vi "Write Next Row (First Column).vi"(8 "error in (no error)":errorcluster, 10 "Next Row":i32, 11 "PQ Result  in":refnum<class "PQ Result.lvclass">) -> (0 "error out":errorcluster, 3 "PQ Result  out":refnum<class "PQ Result.lvclass">)   [LabVIEW 2013, in "PQ Result.lvclass"]
uses:
  PQ Result.lvclass
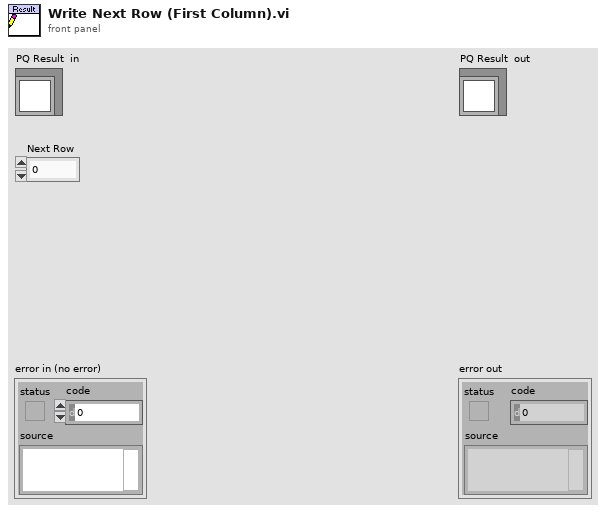
[diagram p1: front panel]
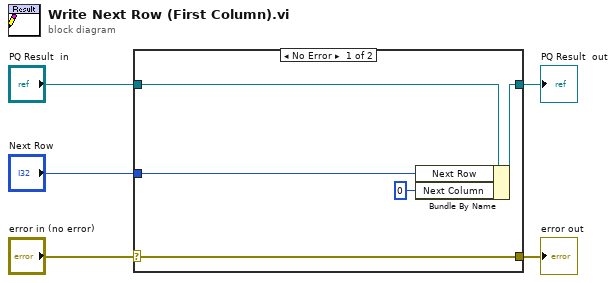
[diagram p0: block diagram]
diagram:
  n1 = case shown="No Error" "error in (no error)" {
    selector: "error in (no error)" -> [w10 w11]
    tunnel: [w10 w11] -> w4
    tunnel: [w8 w12] -> w2
    tunnel: "PQ Result  in" -> [w9 w12]
    tunnel: "Next Row" -> [w7 _]
    frame No Error {
      n2 = Bundle By Name(cluster=w9, "Next Row"=w7, "Next Column"=0) -> (w8:refnum<class "PQ Result.lvclass">)
    }
    frame Error {
    }
  }
  "error out" <- w4
  "PQ Result  out" <- w2
